vi "Run.vi"(8 "error in (no error)":errorcluster caption="entrée d'erreur (pas d'erreur)", 9 "labels_pred":string[][](array[string]), 10 "labels_true":string[][](array[string]), 11 "Normalized_Mutual_Info_Score.lvclass":refnum<class "Normalized_Mutual_Info_Score.lvclass">) -> (0 "error out":errorcluster caption="sortie d'erreur", 2 "String Data":string, 3 "Normalized_Mutual_Info_Score.lvclass":refnum<class "Normalized_Mutual_Info_Score.lvclass">)   [LabVIEW 2020, in "Normalized_Mutual_Info_Score.lvclass"]
doc: "Returns : \n\n- nmi : float\nscore between 0.0 and 1.0. 1.0 stands for perfectly complete labeling"
uses:
  Normalized_Mutual_Info_Score.lvclass
  Normalized_Mutual_Info_Score.lvclass/Normalized_Mutual_Info_Score.ctl
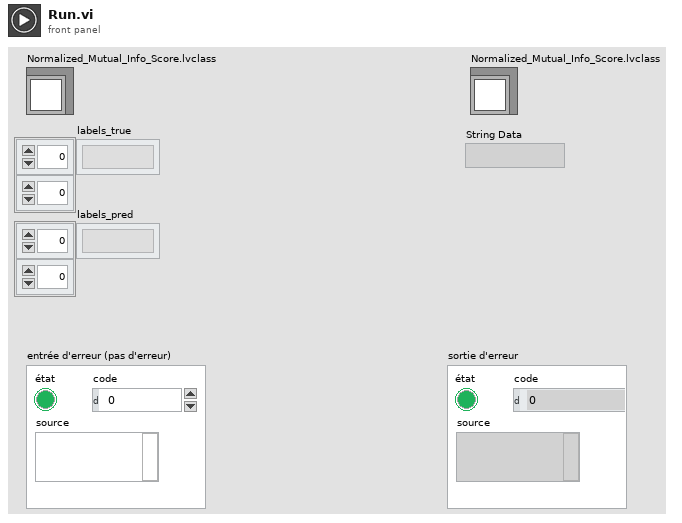
[diagram p1: front panel]
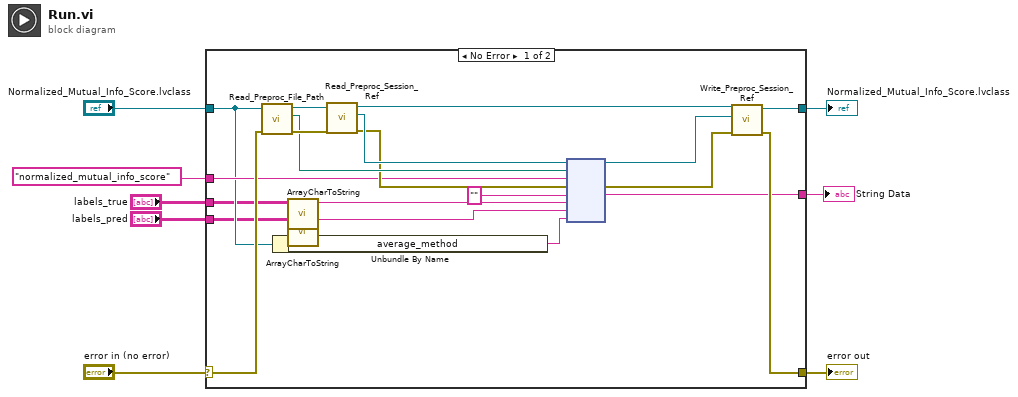
[diagram p0: block diagram]
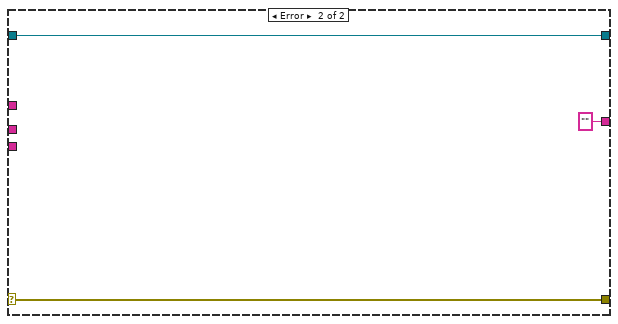
[diagram p2: hidden frame]
diagram:
  n1 = case shown="No Error" "error in (no error)" {
    selector: "error in (no error)" -> [w17 w31]
    tunnel: [w18 w31] -> w7
    tunnel: [w19 w30] -> w5
    tunnel: "Normalized_Mutual_Info_Score.lvclass" -> [w14 w30]
    tunnel: "normalized_mutual_info_score" -> [w16 _]
    tunnel: [w15 ""] -> w4
    tunnel: "labels_true" -> [w12 _]
    tunnel: "labels_pred" -> [w11 _]
    frame No Error {
      n2 = call-dynamic "Read_Preproc_File_Path.vi"("error in (no error)"=w17, "Python in"=w14) -> ("error out"=w27:errorcluster, "File_Path"=w26:path, "Python out"=w28:refnum<class "Normalized_Mutual_Info_Score.lvclass">)  [unwired: 7 in]
      n3 = Unbundle By Name(w14) -> ("average_method"=w13:string)
      n4 = call "ArrayCharToString.vi"("TAB"=w12) -> ("Instruction"=w10:string)  [unwired: 10 in]
      n5 = call "ArrayCharToString.vi"("TAB"=w11) -> ("Instruction"=w9:string)  [unwired: 10 in]
      n6 = call-dynamic "Read_Preproc_Session_Ref.vi"("error in (no error)"=w27, "Python in"=w28) -> ("error out"=w24:errorcluster, "Session_ref"=w25:refnum<k35>, "Python out"=w23:refnum<class "Normalized_Mutual_Info_Score.lvclass">)  [unwired: 7 in]
      n7 = node(w25, w26, w16, w24, "", w10, w9, w13) -> (w21:refnum<k35>, w22:errorcluster, w15:string)  [unwired: 3 in, 2 out]
      n8 = call-dynamic "Write_Preproc_Session_Ref.vi"("error in (no error)"=w22, "Session_ref"=w21, "Python in"=w23) -> ("error out"=w18:errorcluster, "Python out"=w19:refnum<class "Normalized_Mutual_Info_Score.lvclass">)  [unwired: 7 in]
    }
    frame Error {
    }
  }
  "error out" <- w7
  "Normalized_Mutual_Info_Score.lvclass" <- w5
  "String Data" <- w4
